vi "Select PID Values.vi"(10 "current field":dbl[unit], 11 "varian in":refnum<class "Varian Magnet.lvclass">) -> (2 "PID output":cluster{"I":dbl, "D":dbl, "P":dbl}, 3 "varian out":refnum<class "Varian Magnet.lvclass">)   [LabVIEW 2009, in "Varian Magnet.lvclass"]
doc: "this returns the appropriate PID settings when the control voltage is 40V...change later to adapt to 30V settings too."
uses:
  Varian Magnet.lvclass
  Varian Magnet.lvclass/Varian Magnet.ctl
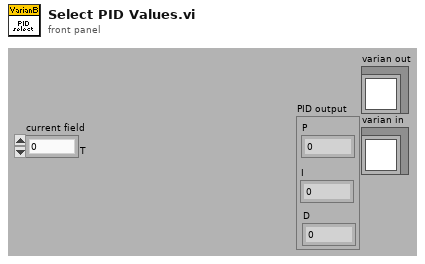
[diagram p1: front panel]
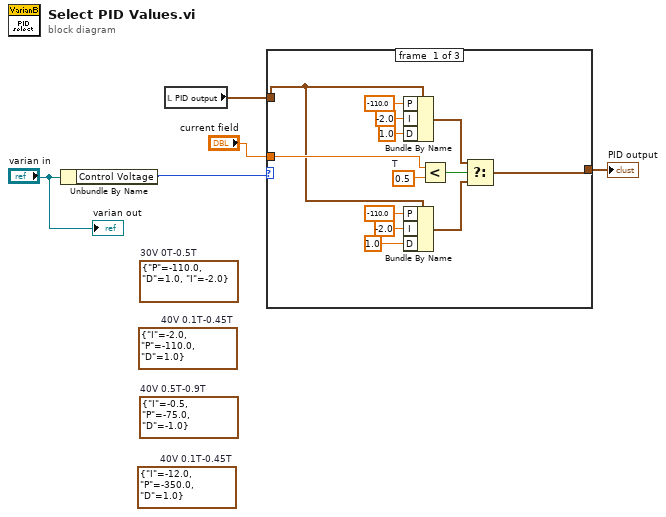
[diagram p0: block diagram]
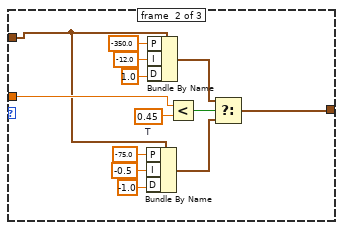
[diagram p2: hidden frame]
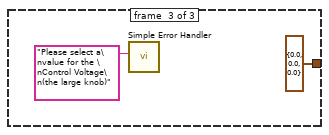
[diagram p3: hidden frame]
diagram:
  (unwired) cluster{"I":dbl, "P":dbl, "D":dbl} {"I"=-12.0, "P"=-350.0, "D"=1.0}  # 40V 0.1T-0.45T
  (unwired) cluster{"I":dbl, "P":dbl, "D":dbl} {"I"=-0.5, "P"=-75.0, "D"=-1.0}  # 40V 0.5T-0.9T
  (unwired) cluster{"I":dbl, "P":dbl, "D":dbl} {"I"=-2.0, "P"=-110.0, "D"=1.0}  # 40V 0.1T-0.45T
  (unwired) cluster{"P":dbl, "D":dbl, "I":dbl} {"P"=-110.0, "D"=1.0, "I"=-2.0}  # 30V 0T-0.5T
  n1 = Unbundle By Name("varian in") -> ("Control Voltage"=w2:enum16{"Please Select a Value", "30V", "40V"})
  n2 = local read "PID output"() -> (w3:cluster{"I":dbl, "D":dbl, "P":dbl})
  n3 = case shown="\"40V\", Default" w2 {
    tunnel: [w15 w20 cluster{"I":dbl, "P":dbl, "D":dbl} {"I"=0.0, "P"=0.0, "D"=0.0} ("40V 0.1T-0.45T")] -> w5
    tunnel: "current field" -> [w16 w29 _]
    tunnel: w3 -> [w12 w22 _]
    frame #0 {
      w18 = dbl[unit] 0.5  # T
      n4 = Bundle By Name(cluster=w12, "P"=-110.0, "I"=-2.0, "D"=1.0) -> (w14:cluster{"I":dbl, "D":dbl, "P":dbl})
      n5 = Bundle By Name(cluster=w12, "P"=-110.0, "I"=-2.0, "D"=1.0) -> (w13:cluster{"I":dbl, "D":dbl, "P":dbl})
      n6 = Less?(x=w16, y=w18) -> (x < y?=w17:bool)
      n7 = Select(t=w14, s=w17, f=w13) -> (s? t:f=w15:cluster{"I":dbl, "D":dbl, "P":dbl})
    }
    frame #1 {
      w31 = dbl[unit] 0.45  # T
      n8 = Bundle By Name(cluster=w22, "P"=-75.0, "I"=-0.5, "D"=-1.0) -> (w21:cluster{"I":dbl, "D":dbl, "P":dbl})
      n9 = Bundle By Name(cluster=w22, "P"=-350.0, "I"=-12.0, "D"=1.0) -> (w28:cluster{"I":dbl, "D":dbl, "P":dbl})
      n10 = Less?(x=w29, y=w31) -> (x < y?=w30:bool)
      n11 = Select(t=w28, s=w30, f=w21) -> (s? t:f=w20:cluster{"I":dbl, "D":dbl, "P":dbl})
    }
    frame #2 {
      n12 = call <vilib>:"Simple Error Handler.vi"("error source (\" \")"="Please select a\nvalue for the \nControl Voltage\n(the large knob)" ("error source (\" \")")) -> ()  [unwired: 4 in, 5 out]
    }
  }
  "PID output" <- w5
  "varian out" <- "varian in"
